vi "Check If Calibration Data Exist_MultiMix.vi"(5 "Set Pressure Cluster":T1, 6 "Water Mix Pressure Group":u8=2, 7 "Mix Sequence Array":bool[][](array[boolean]), 8 "Water Mix Valve":u16(ring)=14 items=["A1", "A2", "A3", "A4", "B1", "B2", "B3", "B4", "B5", "B6", "B7", "B8", "A5", "A6", "A7", "A8"], 9 "Possible Water Mix Ratios":dbl[](array[numeric]), 10 "Pressure Group":enum16{"1", "2", "3", "4"}[](array[ring])=[enum."3", enum."3", enum."3", enum."3", enum."4", enum."4", enum."4", enum."4", enum."1", enum."1", enum."1", enum."1", enum."1"], 11 "Calibration Refs":T2) -> (1 "Calibration Data Exists?":bool, 2 "Psequence":dbl[][](array[numeric]))   [LabVIEW 2016]
uses:
  <vilib>/imath/engines/lvmath2/RunTimeEngine/Managers/WorkSpace/UID Generator.vi
  <vilib>/imath/engines/lvmath2/RunTimeEngine/BuiltInFunctions/any/NIMS_any(GM).vi
  <vilib>/imath/engines/lvmath2/RunTimeEngine/VariableToken/Support/NIMS_Matrix Boolean Index to I32 Index.vi
  <vilib>/imath/engines/lvmath2/RunTimeEngine/IndexRead/NIMS V(V).vi
  <instcachedir>/0/NIMS V(V)_298D9CB7BFEB42B8BC8D9C3C28AE8C70.lvgen/NIMS V(V)_298D9CB7BFEB42B8BC8D9C3C28AE8C70_004.vi
  <vilib>/imath/engines/lvmath2/RunTimeEngine/BuiltInFunctions/sets_unique/NIMS_sets_unique(GV).vi
  <instcachedir>/0/NIMS_sets_unique(GV)_BC60CBD939E647F382369330BF9EA64D.lvgen/NIMS_sets_unique(GV)_BC60CBD939E647F382369330BF9EA64D_007.vi
  <vilib>/imathl/engines/lvmath/Functions/Error Handling/Create Error.vi
  <vilib>/imath/engines/lvmath2/RunTimeEngine/BuiltInFunctions/sets_intersect/NIMS_sets_intersect(GV2).vi
  <instcachedir>/0/NIMS_sets_intersect(GV2)_74AAA1A47D014705AAA1ED31FAC0AF67.lvgen/NIMS_sets_intersect(GV2)_74AAA1A47D014705AAA1ED31FAC0AF67_008.vi
  <vilib>/imath/engines/lvmath2/RunTimeEngine/BuiltInFunctions/size/NIMS_I32=size(GM,I32).vi
  <instcachedir>/0/NIMS_I32=size(GM,I32)_9B6975FE2A37478D9DF1A6A9597B9E6B.lvgen/NIMS_I32=size(GM,I32)_9B6975FE2A37478D9DF1A6A9597B9E6B_005.vi
  <vilib>/imath/engines/lvmath2/RunTimeEngine/BuiltInFunctions/length/NIMS_length(GV).vi
  <instcachedir>/0/NIMS_length(GV)_08A3D13377FD4E4B96F5795FBF3698FA.lvgen/NIMS_length(GV)_08A3D13377FD4E4B96F5795FBF3698FA_002.vi
  <vilib>/imath/engines/lvmath2/RunTimeEngine/RangeToken/NIMS_Range_R2 - Integer.vi
  <instcachedir>/0/NIMS_Range_R2 - Integer_416A044C4F024DBE8E97DA138CB3186F.lvgen/NIMS_Range_R2 - Integer_416A044C4F024DBE8E97DA138CB3186F_000.vi
  <vilib>/imath/engines/lvmath2/RunTimeEngine/CommandStatement/MC_CommandStatement_break.vi
  <vilib>/imath/engines/lvmath2/RunTimeEngine/IndexRead/NIMS V(S).vi
  <instcachedir>/0/NIMS V(S)_0488751826AF41519A22953C041130DC.lvgen/NIMS V(S)_0488751826AF41519A22953C041130DC_002.vi
  <instcachedir>/0/NIMS V(S)_0488751826AF41519A22953C041130DC.lvgen/NIMS V(S)_0488751826AF41519A22953C041130DC_000.vi
  <vilib>/imath/engines/lvmath2/RunTimeEngine/IndexReplace/NIMS M($,S)=S.vi
  <instcachedir>/0/NIMS M($,S)=S_A0423FE00DA742AC8AE5C29177BBA576.lvgen/NIMS M($,S)=S_A0423FE00DA742AC8AE5C29177BBA576_000.vi
  <vilib>/imath/engines/lvmath2/RunTimeEngine/ErrorHandling/NIMS_Create Error From Enums.vi
  <vilib>/imath/engines/lvmath2/RunTimeEngine/VariableToken/NIMS_VariableToken_CondDefinedDefinedByReplace.vi
  <instcachedir>/0/NIMS_VariableToken_CondDefinedDefinedByReplace_D162CFFC24174562A9FEA619A91E1A56.lvgen/NIMS_VariableToken_CondDefinedDefinedByReplace_D162CFFC24174562A9FEA619A91E1A56_004.vi
  <vilib>/imath/engines/lvmath2/RunTimeEngine/IndexRead/NIMS M(S,$).vi
  <instcachedir>/0/NIMS M(S,$)_F24F360562DE41D8BE234322A2E15C65.lvgen/NIMS M(S,$)_F24F360562DE41D8BE234322A2E15C65_002.vi
  <vilib>/imath/engines/lvmath2/RunTimeEngine/BuiltInFunctions/findnz/NIMS_[1o]_findnz(GRowV).vi
  <instcachedir>/0/NIMS_[1o]_findnz(GRowV)_656056C849EF4762B1F0843BDDDEF2FF.lvgen/NIMS_[1o]_findnz(GRowV)_656056C849EF4762B1F0843BDDDEF2FF_000.vi
  <vilib>/imath/engines/lvmath2/RunTimeEngine/IndexReplace/NIMS V(S)=S.vi
  <instcachedir>/0/NIMS V(S)=S_5B9D821375184D3582A2146CD1A04ED7.lvgen/NIMS V(S)=S_5B9D821375184D3582A2146CD1A04ED7_003.vi
  <instcachedir>/0/NIMS_VariableToken_CondDefinedDefinedByReplace_D162CFFC24174562A9FEA619A91E1A56.lvgen/NIMS_VariableToken_CondDefinedDefinedByReplace_D162CFFC24174562A9FEA619A91E1A56_005.vi
  <instcachedir>/0/NIMS V(S)=S_5B9D821375184D3582A2146CD1A04ED7.lvgen/NIMS V(S)=S_5B9D821375184D3582A2146CD1A04ED7_000.vi
  <vilib>/imath/engines/lvmath2/RunTimeEngine/BuiltInFunctions/round/NIMS_round(DBL-V).vi
  <vilib>/imath/engines/lvmath2/RunTimeEngine/BuiltInFunctions/round/NIMS_round(DBL-S).vi
  <vilib>/imath/engines/lvmath2/RunTimeEngine/RunTimeType/NIMS_RunTimeType_From StrictType (excl LVString).vi
  <instcachedir>/0/NIMS_RunTimeType_From StrictType (excl LVString)_CEE1C65A8F1B491DB327E5E54E5E7674.lvgen/NIMS_RunTimeType_From StrictType (excl LVString)_CEE1C65A8F1B491DB327E5E54E5E7674_000.vi
  <vilib>/imath/engines/lvmath2/RunTimeEngine/RunTimeType/NIMS_RunTimeType_Set Source Original Bool.vi
  <vilib>/imath/engines/lvmath2/RunTimeEngine/LocalVariableDefStatement/MC_LocalVariableDefStatement_Display.vi
  <vilib>/imath/engines/lvmath2/RunTimeEngine/BitwiseOperatorToken/NIMS_Bitwise_Operator_And.vi
  <instcachedir>/0/NIMS_Bitwise_Operator_And_FD93B025054444799547119B3AA78300.lvgen/NIMS_Bitwise_Operator_And_FD93B025054444799547119B3AA78300_001.vi
  <vilib>/imath/engines/lvmath2/RunTimeEngine/BuiltInFunctions/any/NIMS_any(GRowV).vi
  <vilib>/imath/engines/lvmath2/RunTimeEngine/VariableToken/Support/NIMS_Vector Boolean Index to I32 Index.vi
  <instcachedir>/0/NIMS V(V)_298D9CB7BFEB42B8BC8D9C3C28AE8C70.lvgen/NIMS V(V)_298D9CB7BFEB42B8BC8D9C3C28AE8C70_002.vi
  <vilib>/imath/engines/lvmath2/RunTimeEngine/IndexReplace/NIMS M(S,S)=V.vi
  <instcachedir>/0/NIMS M(S,S)=V_15AD8FB2967743539B9C55B25408BFD2.lvgen/NIMS M(S,S)=V_15AD8FB2967743539B9C55B25408BFD2_000.vi
  <vilib>/imath/engines/lvmath2/RunTimeEngine/Managers/SymbolTable/Clear UID.vi
  <vilib>/imath/engines/lvmath2/RunTimeEngine/NodeEndStatement/NIMS_NodeEndStatement_Output.vi
  <instcachedir>/0/NIMS_NodeEndStatement_Output_53EC0D466D134D7ABD903AC30B43404B.lvgen/NIMS_NodeEndStatement_Output_53EC0D466D134D7ABD903AC30B43404B_002.vi
  <instcachedir>/0/NIMS_NodeEndStatement_Output_53EC0D466D134D7ABD903AC30B43404B.lvgen/NIMS_NodeEndStatement_Output_53EC0D466D134D7ABD903AC30B43404B_010.vi
  <vilib>/imath/engines/lvmath2/RunTimeEngine/ErrorHandling/NIMS_Finalize Error.vi
  <vilib>/imath/engines/lvmath2/RunTimeEngine/Managers/SymbolTable/NIMS_WorkSpace.lvlib
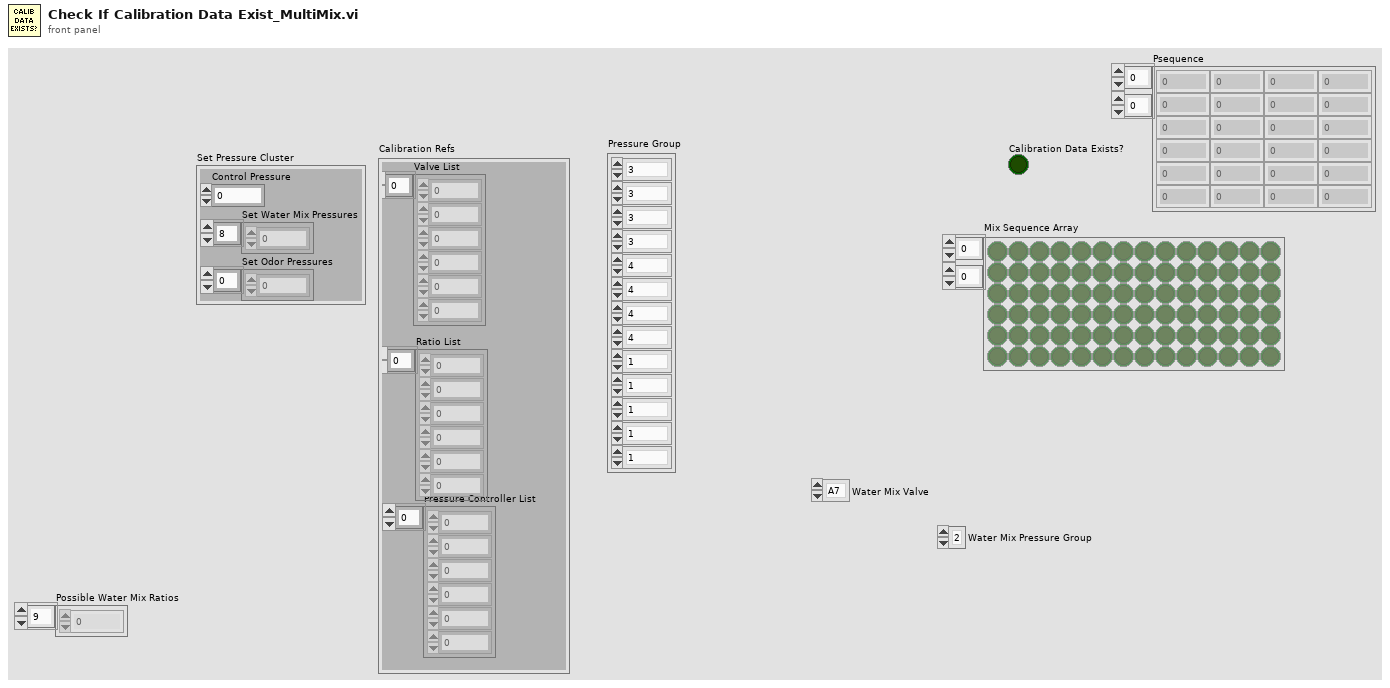
[diagram p1: front panel]
types:
  T1 = cluster{"Control Pressure":dbl, "Set Water Mix Pressures":dbl[], "Set Odor Pressures":dbl[]}
  T2 = cluster{"Pressure Controller List":u8[], "Ratio List":dbl[], "Valve List":u16[]}
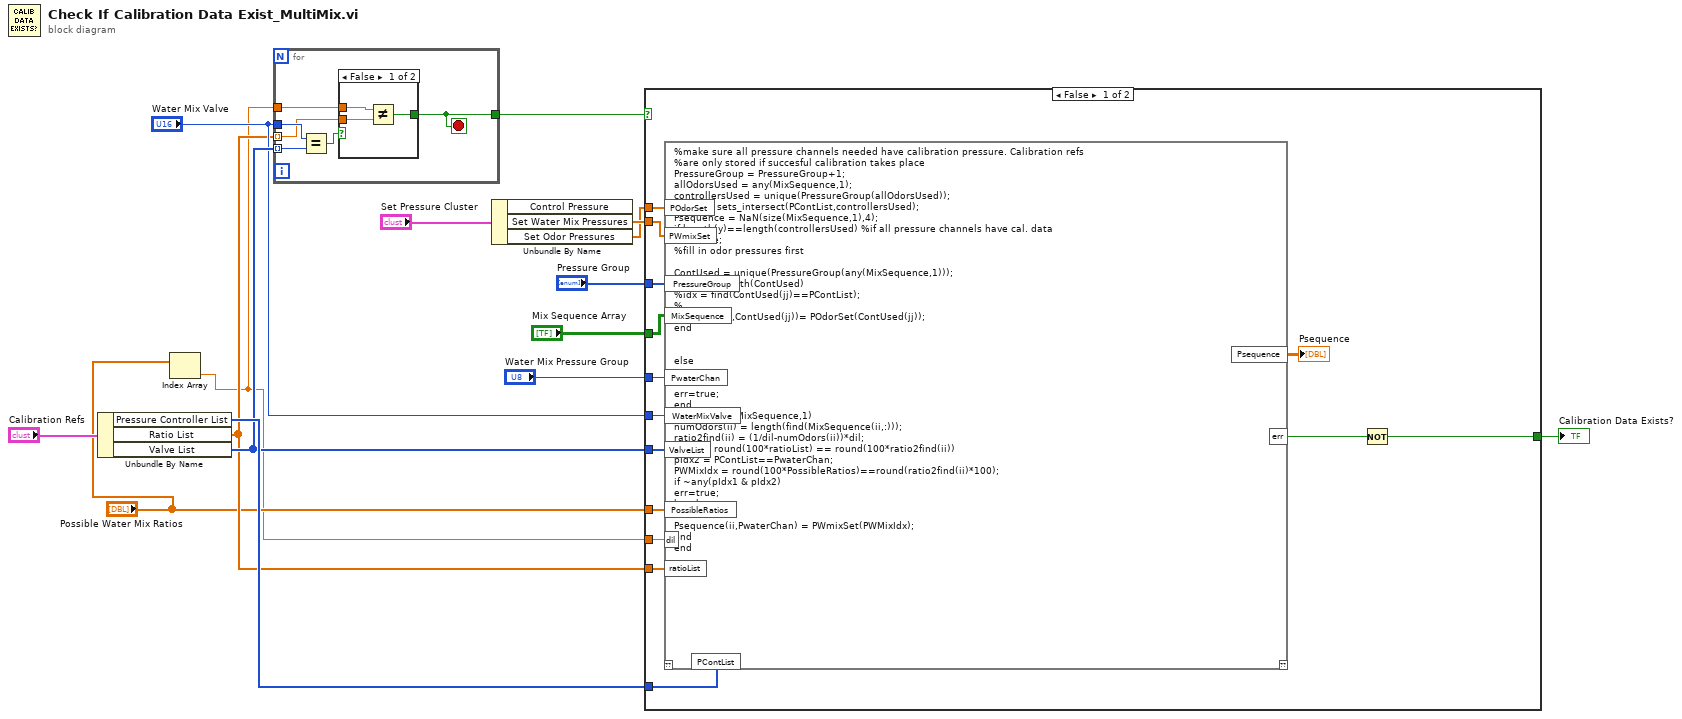
[diagram p0: block diagram]
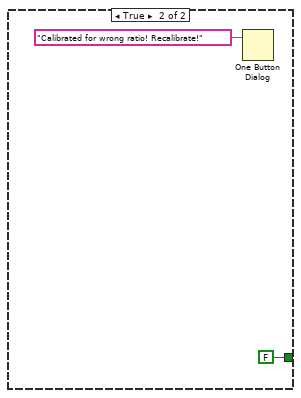
[diagram p2: hidden frame]
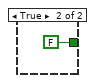
[diagram p3: hidden frame]
diagram:
  n1 = Unbundle By Name("Calibration Refs") -> ("Pressure Controller List"=w12:u8[], "Ratio List"=w5:dbl[], "Valve List"=w11:u16[])
  n2 = Index Array(array="Possible Water Mix Ratios") -> (element=w1:dbl)  [unwired: 1 in]
  n3 = for {
    tunnel: w11 -> [w20] mode=indexing
    tunnel: "Water Mix Valve" -> [w21]
    tunnel: w5 -> [w17] mode=indexing
    tunnel: w1 -> [w18]
    tunnel: [w16] -> w9
    stop <- w16 stop-if-true
    n4 = Equal?(x=w21, y=w20) -> (x = y?=w19:bool)
    n5 = case shown="False" w19 {
      tunnel: w18 -> [w24 _]
      tunnel: w17 -> [w23 _]
      tunnel: [w22 FALSE] -> w16
      frame False {
        n6 = Not Equal?(x=w24, y=w23) -> (x != y?=w22:bool)
      }
      frame True {
      }
    }
  }
  n7 = Unbundle By Name("Set Pressure Cluster") -> ("Set Water Mix Pressures"=w4:dbl[], "Set Odor Pressures"=w3:dbl[])  [unwired: 1 out]
  n8 = case shown="False" w9 {
    tunnel: "Mix Sequence Array" -> [w39 _]
    tunnel: w4 -> [w38 _]
    tunnel: "Pressure Group" -> [w37 _]
    tunnel: w12 -> [w36 _]
    tunnel: w11 -> [w35 _]
    tunnel: "Water Mix Valve" -> [w34 _]
    tunnel: "Water Mix Pressure Group" -> [w32 _]
    tunnel: w1 -> [w31 _]
    tunnel: w5 -> [w30 _]
    tunnel: [w28 FALSE ("err")] -> w7
    tunnel: w3 -> [w27 _]
    tunnel: "Possible Water Mix Ratios" -> [w26 _]
    frame False {
      n9 = mathscript code="%make sure all pressure channels needed have calibration pressure. Calibration refs\n%are only stored if succesful calibration takes place\nPressureGroup = PressureGroup+1;\nallOdorsUsed = any(MixSequence,1);\ncontrollersUsed = unique(PressureGroup(allOdorsUsed));\n[x,y,z] = sets_intersect(PContList,controllersUsed);\nPsequence = NaN(size(MixSequence,1),4);\nif length(y)==length(controllersUsed) %if all pressure channels have cal. data\nerr=false;\n%fill in odor pressures first\n\nContUsed = unique(PressureGroup(any(MixSequence,1)));\nfor jj = 1:length(ContUsed)\n%idx = find(ContUsed(jj)==PContList);\n% \nPsequence(:,ContUsed(jj))= POdorSet(ContUsed(jj));\nend\n\n\nelse\n\n\nerr=true;\nend\nfor ii=1:size(MixSequence,1)\nnumOdors(ii) = length(find(MixSequence(ii,:)));\nratio2find(ii) = (1/dil-numOdors(ii))*dil;\npIdx1 = round(100*ratioList) == round(100*ratio2find(ii))\npIdx2 = PContList==PwaterChan;\nPWMixIdx = round(100*PossibleRatios)==round(ratio2find(ii)*100);\nif ~any(pIdx1 & pIdx2)\nerr=true;\nbreak\nelse\nPsequence(ii,PwaterChan) = PWmixSet(PWMixIdx);\nend\nend"("PressureGroup"=w37, "MixSequence"=w39, "WaterMixValve"=w34, "ValveList"=w35, "PContList"=w36, "PWmixSet"=w38, "PwaterChan"=w32, "dil"=w31, "ratioList"=w30, "POdorSet"=w27, "PossibleRatios"=w26) -> ("Psequence"=→"Psequence":dbl[][], "err"=w29:bool)  [unwired: 1 in, 1 out]
      n10 = Not(x=w29) -> (.not. x?=w28:bool)
    }
    frame True {
      n11 = One Button Dialog(message="Calibrated for wrong ratio! Recalibrate!") -> ()  [unwired: 1 in, 1 out]
    }
  }
  "Calibration Data Exists?" <- w7
